vi "露点温度.vi"(1 "水蒸気圧":dbl) -> (0 "露点温度":dbl)   [LabVIEW 2014]
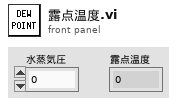
[diagram p1: front panel]
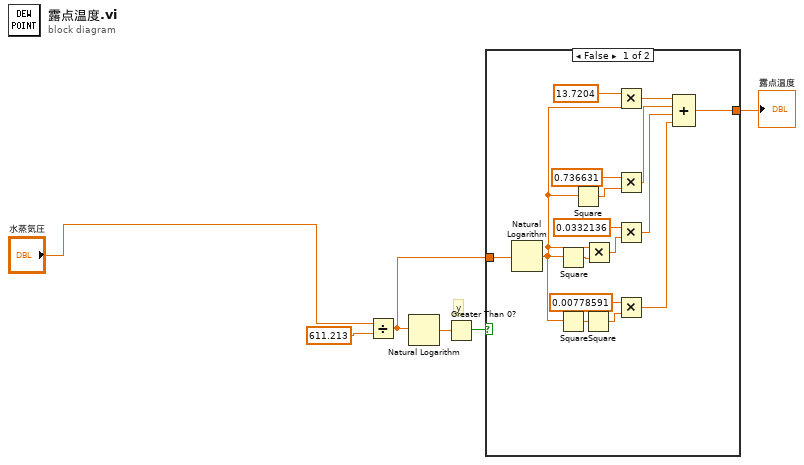
[diagram p0: block diagram]
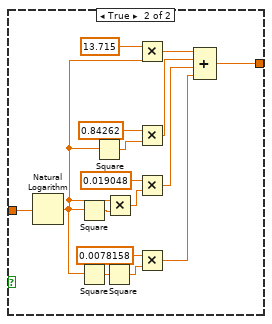
[diagram p2: hidden frame]
diagram:
  # "y"
  n1 = Divide(x="水蒸気圧", y=611.213 ("x")) -> (x/y=w3:dbl)
  n2 = Natural Logarithm(1:w3) -> (0:w2:dbl)
  n3 = Greater Than 0?(x=w2) -> (x > 0?=w1:bool)
  n4 = case shown="FALSE" w1 {
    tunnel: w3 -> [w9 w37]
    tunnel: [w10 w25] -> w4
    frame False {
      n5 = Natural Logarithm(1:w9) -> (0:w20:dbl)
      n6 = Square(x=w20) -> (x^2=w15:dbl)
      n7 = Square(x=w20) -> (x^2=w19:dbl)
      n8 = Square(x=w20) -> (x^2=w13:dbl)
      n9 = Square(x=w19) -> (x^2=w18:dbl)
      n10 = Multiply(x=w20, y=w15) -> (x*y=w16:dbl)
      n11 = Multiply(x=13.7204, y=w20) -> (x*y=w21:dbl)
      n12 = Multiply(x=0.736631, y=w13) -> (x*y=w22:dbl)
      n13 = Multiply(x=0.0332136, y=w16) -> (x*y=w8:dbl)
      n14 = Multiply(x=0.00778591, y=w18) -> (x*y=w7:dbl)
      n15 = Compound Arithmetic op=ADD(w21, w22, w8, w7) -> (w10:dbl)
    }
    frame True {
      n16 = Natural Logarithm(1:w37) -> (0:w28:dbl)
      n17 = Square(x=w28) -> (x^2=w33:dbl)
      n18 = Square(x=w28) -> (x^2=w29:dbl)
      n19 = Square(x=w28) -> (x^2=w35:dbl)
      n20 = Square(x=w29) -> (x^2=w30:dbl)
      n21 = Multiply(x=w28, y=w33) -> (x*y=w32:dbl)
      n22 = Multiply(x=13.715, y=w28) -> (x*y=w27:dbl)
      n23 = Multiply(x=0.84262, y=w35) -> (x*y=w26:dbl)
      n24 = Multiply(x=0.019048, y=w32) -> (x*y=w24:dbl)
      n25 = Multiply(x=0.0078158, y=w30) -> (x*y=w23:dbl)
      n26 = Compound Arithmetic op=ADD(w27, w26, w24, w23) -> (w25:dbl)
    }
  }
  "露点温度" <- w4
